vi "AllPartInitialization_DL.vi"(8 "error in (no error)":errorcluster, 10 "AllPartInfoArray":T1=[{"PartName"="", "NumberOfRacks"=0, "MeasurementIDsArray"=[], "MeasurementNamesArray"=[], "SpecValuesArray"=[]}], 11 "DataLogger in":refnum<class "DataLogger.lvclass">) -> (0 "error out":errorcluster, 3 "DataLogger out":refnum<class "DataLogger.lvclass">)   [LabVIEW 2019, in "DataLogger.lvclass"]
uses:
  DataLogger.lvclass
  Common/Controls/AllPartInfo.ctl
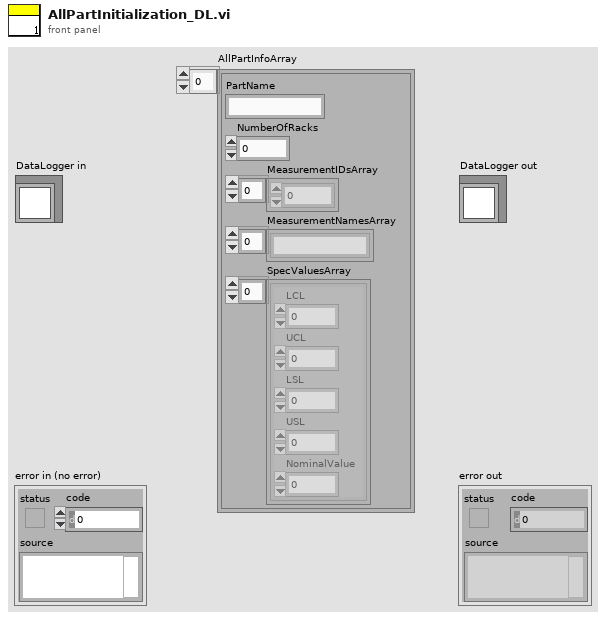
[diagram p1: front panel]
types:
  T1 = typedef "AllPartInfo.ctl" = cluster{"PartName":string, "NumberOfRacks":u8, "MeasurementIDsArray":u16[], "MeasurementNamesArray":string[], "SpecValuesArray":cluster{"LCL":dbl, "UCL":dbl, "LSL":dbl, "USL":dbl, "NominalValue":dbl}[]}[]
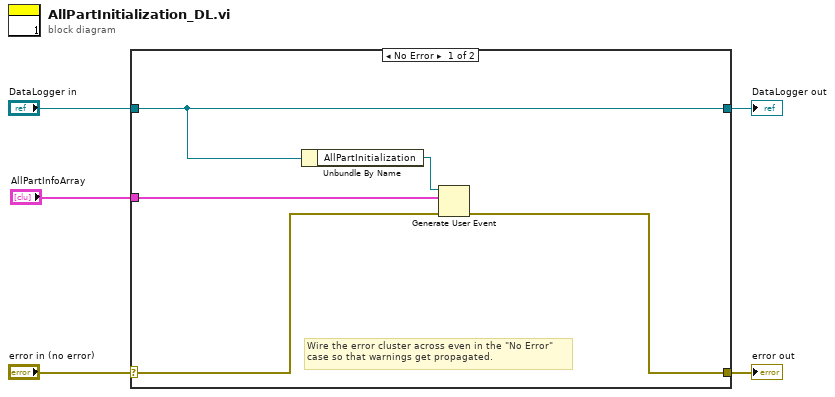
[diagram p0: block diagram]
diagram:
  n1 = case shown="No Error" "error in (no error)" {
    selector: "error in (no error)" -> [w9 w12]
    tunnel: [w8 w12] -> w4
    tunnel: [w7 w11] -> w2
    tunnel: "DataLogger in" -> [w7 w11]
    tunnel: "AllPartInfoArray" -> [w10 _]
    frame No Error {
      # "Wire the error cluster across even in the \"No Error\"\ncase so that warnings get propagated."
      n2 = Unbundle By Name(w7) -> ("AllPartInitialization"=w6:refnum<user-event>)
      n3 = Generate User Event(user event=w6, event data cluster=w10, error in=w9) -> (error out=w8:errorcluster)  [unwired: 1 in, 1 out]
    }
    frame Error {
    }
  }
  "error out" <- w4
  "DataLogger out" <- w2
